vi "Interpolate pockels cell.vi"(8 "no of planes":dbl, 11 "data in":dbl[][](array[numeric])) -> (3 "interpolated data out":dbl[][](array[numeric]))   [LabVIEW 2012]
doc: "SciScan 1.2 160622\nDetermines the following types of interpolation: linear, polynomial, spline, and rational. You can enter the data on the front panel or read it from a file.\n\nNote: You must have the LabVIEW Full or Professional Development Systems to run this example."
uses:
  <vilib>/gmath/NI_Gmath.lvlib
panel:
  out "Waveform Graph":dbl[][](graph)
  out "Waveform Graph 2":dbl[][](graph)
  # "x"
  # "y"
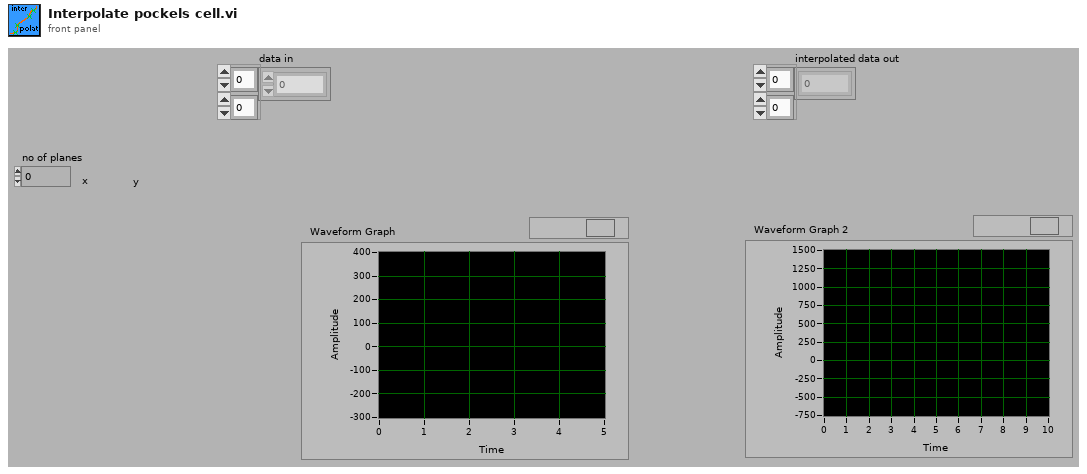
[diagram p1: front panel]
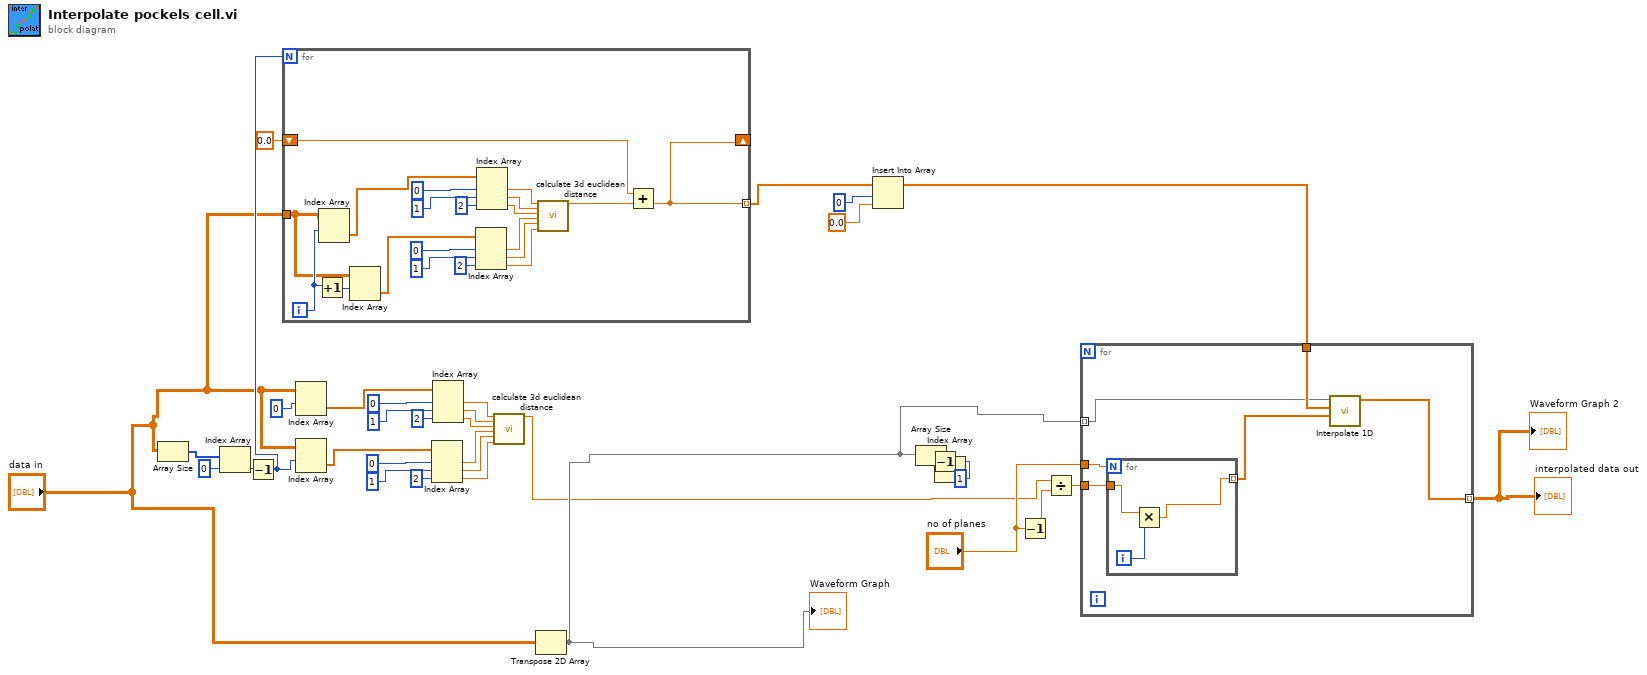
[diagram p0: block diagram]
diagram:
  n1 = Array Size(array="data in") -> (size(s)=w25:i32[])
  n2 = Index Array(array=w25, index=0) -> (element=w23:i32)
  n3 = Decrement(x=w23) -> (x-1=w7:i32)
  n4 = for {
    N: w7 -> [_]
    tunnel: "data in" -> [w53]
    tunnel: [w36] -> w5 mode=indexing
    shift-right: [w36] -> _
    shift-left: 0.0 ("euclid dist") -> [w35]
    i -> [w54]
    n5 = Increment(x=w54) -> (x+1=w52:i32)
    n6 = Index Array(array=w53, index (row)=w54) -> (element=w39:dbl[])  [unwired: 1 in]
    n7 = Index Array(array=w53, index (row)=w52) -> (element=w38:dbl[])  [unwired: 1 in]
    n8 = Index Array(array=w38, index #1=0 ("index"), index #2=1 ("index"), index #3=2 ("index")) -> (element #1=w49:dbl, element #2=w50:dbl, element #3=w51:dbl)
    n9 = Index Array(array=w39, index #1=0 ("index"), index #2=1 ("index"), index #3=2 ("index")) -> (element #1=w46:dbl, element #2=w47:dbl, element #3=w48:dbl)
    n10 = call "calculate 3d euclidean distance.vi"("x1"=w46, "y1"=w47, "z1"=w48, "x2"=w49, "y2"=w50, "z2"=w51) -> ("euclid dist"=w37:dbl)  [unwired: 13 in]
    n11 = Add(x=w35, y=w37) -> (x+y=w36:dbl)
  }
  n12 = Index Array(array="data in", index (row)=0 ("disabled index (col)")) -> (element=w22:dbl[])  [unwired: 1 in]
  n13 = Index Array(array="data in", index (row)=w7) -> (element=w15:dbl[])  [unwired: 1 in]
  n14 = Index Array(array=w15, index #1=0 ("index"), index #2=1 ("index"), index #3=2 ("index")) -> (element #1=w11:dbl, element #2=w10:dbl, element #3=w9:dbl)
  n15 = Index Array(array=w22, index #1=0 ("index"), index #2=1 ("index"), index #3=2 ("index")) -> (element #1=w14:dbl, element #2=w13:dbl, element #3=w12:dbl)
  n16 = call "calculate 3d euclidean distance.vi"("x1"=w14, "y1"=w13, "z1"=w12, "x2"=w11, "y2"=w10, "z2"=w9) -> ("euclid dist"=w8:dbl)  [unwired: 13 in]
  n17 = Transpose 2D Array(2D array="data in") -> (transposed array=w34:dbl[][])
  "Waveform Graph" <- w34
  n18 = Insert Into Array(array=w5, index=0, new element=0.0 ("new element/subarray")) -> (w2:dbl[])
  n19 = Array Size(array=w34) -> (size(s)=w28:i32[])
  n20 = Index Array(array=w28, index=1) -> (element=w30:i32)
  n21 = Decrement(x=w30) -> ()  [unwired: 1 out]
  n22 = Decrement(x="no of planes") -> (x-1=w31:dbl)
  n23 = Divide(x=w8, y=w31) -> (x/y=w32:dbl)
  n24 = for {
    tunnel: w34 -> [w56] mode=indexing
    tunnel: "no of planes" -> [w60]
    tunnel: w32 -> [w59]
    tunnel: [w55] -> w33 mode=indexing
    tunnel: w2 -> [w57]
    n25 = for {
      N: w60 -> [_]
      tunnel: w59 -> [w62]
      tunnel: [w61] -> w58 mode=indexing
      i -> [w63]
      n26 = Multiply(x=w62, y=w63) -> (x*y=w61:dbl)
    }
    n27 = call <vilib>:"Interpolate 1D.vi"("xi"=w58, "X"=w57, "Y"=w56) -> ("yi"=w55:dbl[])  [unwired: 6 in, 2 out]
  }
  "interpolated data out" <- w33
  "Waveform Graph 2" <- w33
